vi "Publish Group Control Page.vi"(7 "LabVIEW Web Service Request":refnum<class "Web Request.lvclass">) -> ()   [LabVIEW 2018]
uses:
  <vilib>/wsapi/Web Request.lvclass
panel:
  # "Use the Web Service Request input terminal to call the VIs on the Web Services palette. Do not remove it from the connector pane unless you don't need access to the palette."
  # "Each additional control wired to the connector pane will be available as an input in the URL. To include an indicator in terminal-mode output (the default setting), it must also be wired to the connector pane."
  # "controls wired to the connector pane of a web resource are essentially local variables for that web resource (vi).\nThey are \"set\" by changing the URL the resource is accessed at, i.e.\ngoing to /CAEN_HV/Config                            will invoke this vi with the default value of ReadBufferView (0).\ngoing to /CAEN_HV/Config/?ReadBufferView=1         will invoke this vi with a ReadBufferView value of 1.\nThese controls can then either change the esp script that is called, to change the page generated, \nor they may be written to ESP variables within the vi, which can then be read within the called .esp script and \nused to render the appropriate html content."
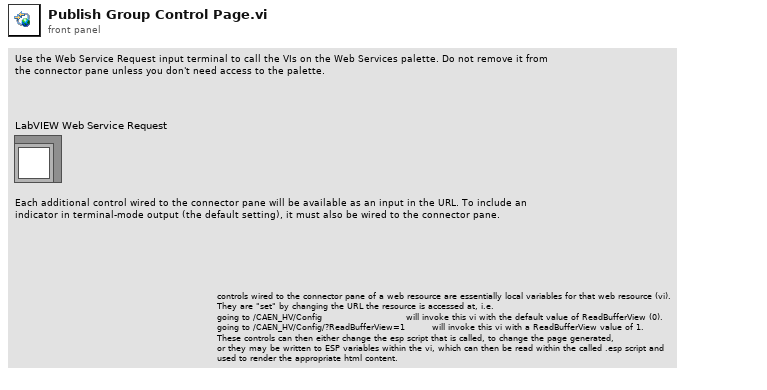
[diagram p1: front panel]
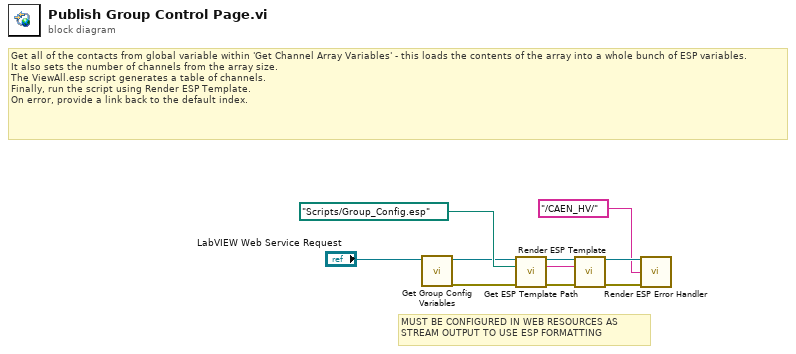
[diagram p0: block diagram]
diagram:
  # "MUST BE CONFIGURED IN WEB RESOURCES AS\nSTREAM OUTPUT TO USE ESP FORMATTING"
  # "Get all of the contacts from global variable within 'Get Channel Array Variables' - this loads the contents of the array into a whole bunch of ESP variables. \nIt also sets the number of channels from the array size. \nThe ViewAll.esp script generates a table of channels. \nFinally, run the script using Render ESP Template. \nOn error, provide a link back to the default index."
  n1 = call "Get Group Config Variables.vi"("LabVIEW Web Service Request"="LabVIEW Web Service Request") -> ("error out"=w1:errorcluster, "LabVIEW Web Service Request out"=w2:refnum<class "Web Request.lvclass">)  [unwired: 9 in]
  n2 = call "Get ESP Template Path.vi"("LabVIEW Web Service Request"=w2, "Relative Template Path"=path "Scripts/Group_Config.esp", "error in (no error)"=w1) -> ("LabVIEW Web Service Request out"=w4:refnum<class "Web Request.lvclass">, "Template Name"=w6:string, "error out"=w7:errorcluster)  [unwired: 10 in]
  n3 = call <vilib>:"Render ESP Template.vi"("LabVIEW Web Service Request"=w4, "espName"=w6, "error in (no error)"=w7) -> ("LabVIEW Web Service Request out"=w9:refnum<class "Web Request.lvclass">, "error out"=w10:errorcluster)  [unwired: 11 in]
  n4 = call "Render ESP Error Handler.vi"("LabVIEW Web Service Request"=w9, "Link"="/CAEN_HV/", "error in (no error)"=w10) -> ()  [unwired: 11 in, 2 out]
